vi "PV HiScroll Status requests.vi"(8 "error in (no error)":errorcluster, 9 "Parameter choice":T1(ring), 10 "Adress of unit":u16=2 min=1 max=999 step=1, 11 "VISA session":refnum<visa-resource-name>) -> (0 "error out":errorcluster, 2 "response (data)":string, 3 "dup VISA session":refnum<visa-resource-name>)   [LabVIEW 2021, in "Pfeiffer Vacuum.lvlib"]
doc: "There are 20 parameters available, only one of which can be enabled at a time. \n\nRemote priority (300)\nError code (303)\nOvertemperature drive (304)\nOvertemperature pump (305)\nTarget speed (308)\nActual speed [Hz] (309)\nDevice current [A] (310)\nOperating hours pump [h] (311)\nSoftware version drive (312)\nMotor voltage [V] (313)\nOperating hours drive [h] (314)\nNominal speed [Hz] (default) (315)\nActual power [W] (316)\nTemperature output stage (324)\nTemperature electronic (326)\nTemperature motor (346)\nDevice designation (349)\nTarget speed (397)\nAcutal speed (398)\nNominal speed (399)\n\nNote: read only VI´s"
uses:
  <instrlib>/Pfeiffer Vacuum/Pfeiffer Vacuum.lvlib
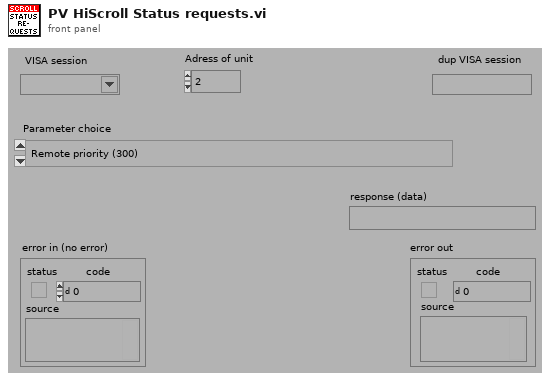
[diagram p1: front panel]
types:
  T1 = enum16{"Remote priority (300)", "Error code (303)", "Overtemperature drive (304)", "Overtemperature pump (305)", "Target speed (308)", "Actual Speed [Hz] (309)", "Intermediate circut current [A] (310)", "Pump operating hours [h] (311)", "Software version of the interface board [312]", "Supply voltage [V] (313)", "Electronic drive unit operating hours [h] (314)", "Nominal speed [Hz] (315)", "Drive power [W] (316)", "Temperature output stage (324)", "Temperature electronic (326)", "Temperature motor (346)", "Device designation (349)", "Target speed (397)", "Acutal speed [rpm] (398)", "Nominal speed [rpm] (399)"}
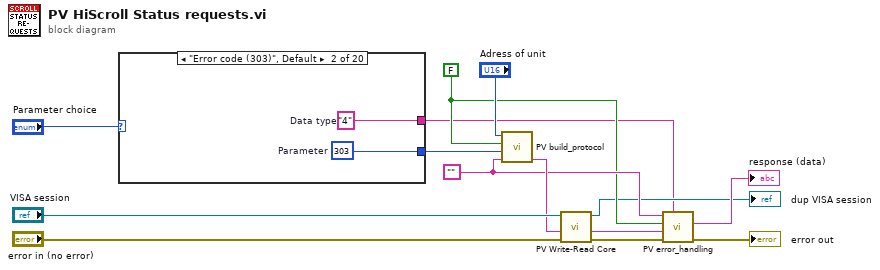
[diagram p0: block diagram]
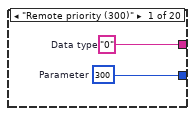
[diagram p2: hidden frame]
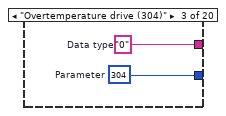
[diagram p3: hidden frame]
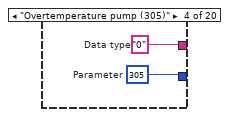
[diagram p4: hidden frame]
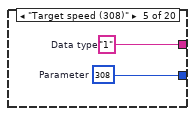
[diagram p5: hidden frame]
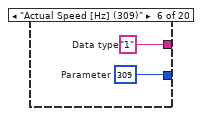
[diagram p6: hidden frame]
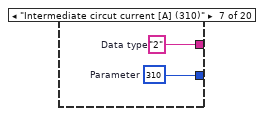
[diagram p7: hidden frame]
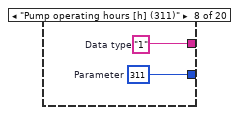
[diagram p8: hidden frame]
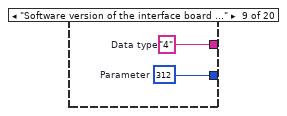
[diagram p9: hidden frame]
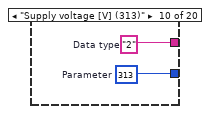
[diagram p10: hidden frame]
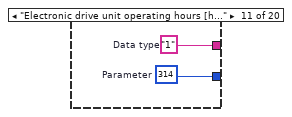
[diagram p11: hidden frame]
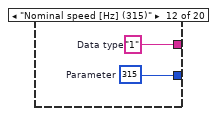
[diagram p12: hidden frame]
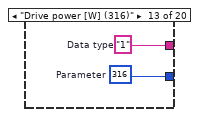
[diagram p13: hidden frame]
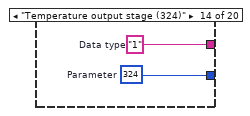
[diagram p14: hidden frame]
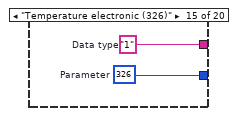
[diagram p15: hidden frame]
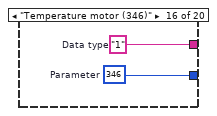
[diagram p16: hidden frame]
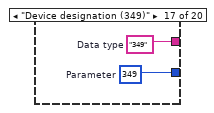
[diagram p17: hidden frame]
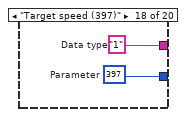
[diagram p18: hidden frame]
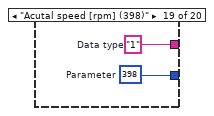
[diagram p19: hidden frame]
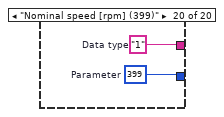
[diagram p20: hidden frame]
diagram:
  w10 = ""
  w9 = FALSE
  n1 = case shown="\"Error code (303)\", Default" "Parameter choice" {
    tunnel: [w15 w17 w19 w22 w23 w26 w28 w30 w32 w34 w36 w38 w40 w41 w43 w45 w48 w50 w52 w54] -> w2
    tunnel: [w16 w18 w20 w21 w24 w25 w27 w29 w31 w33 w35 w37 w39 w42 w44 w46 w47 w49 w51 w53] -> w1
    frame "Remote priority (300)" {
      w15 = "0"  # Data type
      w16 = 300  # Parameter
    }
    frame "Error code (303)", Default {
      w17 = "4"  # Data type
      w18 = 303  # Parameter
    }
    frame "Overtemperature drive (304)" {
      w19 = "0"  # Data type
      w20 = 304  # Parameter
    }
    frame "Overtemperature pump (305)" {
      w21 = 305  # Parameter
      w22 = "0"  # Data type
    }
    frame "Target speed (308)" {
      w23 = "1"  # Data type
      w24 = 308  # Parameter
    }
    frame "Actual Speed [Hz] (309)" {
      w25 = 309  # Parameter
      w26 = "1"  # Data type
    }
    frame "Intermediate circut current [A] (310)" {
      w27 = 310  # Parameter
      w28 = "2"  # Data type
    }
    frame "Pump operating hours [h] (311)" {
      w29 = 311  # Parameter
      w30 = "1"  # Data type
    }
    frame "Software version of the interface board [312]" {
      w31 = 312  # Parameter
      w32 = "4"  # Data type
    }
    frame "Supply voltage [V] (313)" {
      w33 = 313  # Parameter
      w34 = "2"  # Data type
    }
    frame "Electronic drive unit operating hours [h] (314)" {
      w35 = 314  # Parameter
      w36 = "1"  # Data type
    }
    frame "Nominal speed [Hz] (315)" {
      w37 = 315  # Parameter
      w38 = "1"  # Data type
    }
    frame "Drive power [W] (316)" {
      w39 = 316  # Parameter
      w40 = "1"  # Data type
    }
    frame "Temperature output stage (324)" {
      w41 = "1"  # Data type
      w42 = 324  # Parameter
    }
    frame "Temperature electronic (326)" {
      w43 = "1"  # Data type
      w44 = 326  # Parameter
    }
    frame "Temperature motor (346)" {
      w45 = "1"  # Data type
      w46 = 346  # Parameter
    }
    frame "Device designation (349)" {
      w47 = 349  # Parameter
      w48 = "349"  # Data type
    }
    frame "Target speed (397)" {
      w49 = 397  # Parameter
      w50 = "1"  # Data type
    }
    frame "Acutal speed [rpm] (398)" {
      w51 = 398  # Parameter
      w52 = "1"  # Data type
    }
    frame "Nominal speed [rpm] (399)" {
      w53 = 399  # Parameter
      w54 = "1"  # Data type
    }
  }
  n2 = call <instrlib>:"PV build_protocol.vi"("Data"=w10, "Parameter-number"=w1, "parameter\nread<->describe"=w9, "Adress"="Adress of unit") -> ("output"=w11:string)  [unwired: 3 in]
  n3 = call <instrlib>:"PV Write-Read Core.vi"("error in"="error in (no error)", "Write data in"=w11, "VISA session"="VISA session") -> ("error out"=w7:errorcluster, "response (data) out"=w8:string, "dup VISA session"=→"dup VISA session":refnum<visa-resource-name>)  [unwired: 2 in]
  n4 = call <instrlib>:"PV error_handling.vi"("Data Typ in"=w2, "error in"=w7, "response (data) in"=w8, "Parameter\nread only<->describe"=w9, "data in"=w10) -> ("error out"=→"error out":errorcluster, "Data out"=→"response (data)":string)  [unwired: 4 in, 1 out]
